vi "Test Errors Are Logged.vi"(8 "error in (no error)":errorcluster, 11 "Test Case In":refnum<class "Error Handler Tests.lvclass">) -> (0 "error out":errorcluster, 3 "Test Case Out":refnum<class "Error Handler Tests.lvclass">)   [LabVIEW 2020, in "Error Handler Tests.lvclass"]
uses:
  Error Handler Tests.lvclass
  C:/Program Files (x86)/National Instruments/LabVIEW 2020/vi.lib/Astemes/LUnit/Test Case.lvclass
  <vilib>/Astemes/LUnit/Test Case.lvclass/Test Case.ctl
  f68d6c05-d397-4b87-971a-b851a749559a.vi
  <vilib>/Astemes/LUnit/Append Pass Result.vi
  <vilib>/Astemes/LUnit/Append Fail Result.vi
  <vilib>/Astemes/LUnit/Compare Variants.vi
  <vilib>/Astemes/LUnit/Describe Comparison.vi
  <vilib>/Astemes/LUnit/Variant to string.vi
  <vilib>/Utility/Data Type/Get Type Information.vi
  <vilib>/Utility/LVClass/Get LV Class Name.vi
  source/User Interface/Error Handler/Error Handler.lvclass
  source/Support/Utilities.lvlib
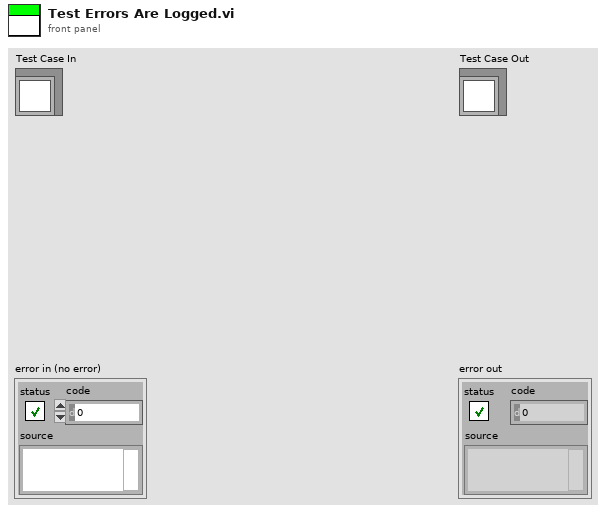
[diagram p1: front panel]
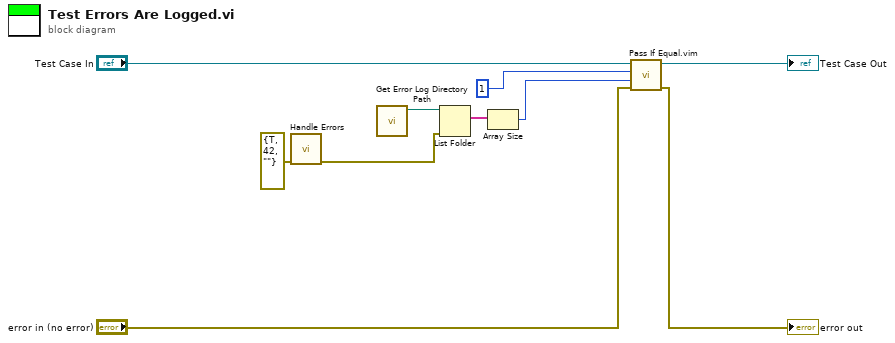
[diagram p0: block diagram]
diagram:
  n1 = call "Handle Errors.vi"("error in (no error)"=errorcluster {"status"=TRUE, "code"=42, "source"=""}) -> ("error out"=w2:errorcluster)  [unwired: 10 in]
  n2 = call "Get Error Log Directory Path.vi"() -> ("Error Log Path"=w6:path)  [unwired: 11 in]
  n3 = List Folder(path=w6, error in=w2) -> (filenames=w5:string[])  [unwired: 2 in, 3 out]
  n4 = Array Size(array=w5) -> (size(s)=w4:i32)
  n5 = call "Pass If Equal.vim"("error in (no error)"="error in (no error)", "Actual"=w4, "Expected"=1 ("size(s)"), "LUnit Test Case In"="Test Case In") -> ("error out"=→"error out":errorcluster, "LUnit Test Case Out"=→"Test Case Out":refnum<class "Error Handler Tests.lvclass">)  [unwired: 6 in]
